vi "Private Global.vi"() -> ()   [LabVIEW 2016, in "Constants.lvlib"]
uses:
  Constants.lvlib
  Typedef/Constants.ctl
  <vilib>/Rock Robotics/SystemInterfaces/DIO/FPGA_DIOPWMChannel.ctl
  <vilib>/Rock Robotics/WPI/Joystick/WPI_JoystickDeviceEnum.ctl
  <vilib>/Rock Robotics/SystemInterfaces/DIO/FPGA_DIOChannel.ctl
  <vilib>/Rock Robotics/SystemInterfaces/spilib/spi_bus.ctl
  <vilib>/Rock Robotics/SystemInterfaces/AI/FPGA_AIChannel.ctl
  <vilib>/Rock Robotics/WPI/Solenoid/WPI_SolenoidChannel.ctl
panel:
  in  "Constants":T1={"Port Layout"={"RightMotorInverted"=FALSE, "LeftMotorInverted"=TRUE, "Left Motors"=enum."PWM 1", "Right Motors"=enum."PWM 0", "Auton List"=["None", "Score Gear Boiler Side", "Score Gear Boiler Side and Shoot", "Score Gear Hopper Side", "Score Gear Center"], "XBOX Port"=enum."USB 0", "Encoder L A"=enum."DIO 0", "Encoder L B"=enum."DIO 1", "Encoder R A"=enum."DIO 2", "Encoder R B"=enum."DIO 3", "L Encoder Inverse"=FALSE, "R Encoder Inverse"=TRUE, "Drive Distance per Count"=0.0490874, "Gyro Bus"=enum."SPI On-Board, CS0", "Fuel Roller 1"=enum."PWM 4", "Front Roller"=enum."PWM 3", "Gear Flipper"=enum."PWM 2", "Climber 1"=enum."PWM 7", "Fuel Roller Invert"=FALSE, "Front Roller Invert"=TRUE, "Gear Flipper Invert"=TRUE, "Climber Invert"=FALSE, "PCM"=1, "Fuel Roller 2"=enum."PWM 5", "Gear Sensor"=enum."AI 0", "Gear Release Fwd"=enum."Solenoid 3", "Gear Release Rvrs"=enum."Solenoid 2", "Fuel Arm Fwd"=enum."Solenoid 4", "Fuel Arm Rvrs"=enum."Solenoid 5", "Shifter Fwrd"=enum."Solenoid 0", "Shifter Rvrs"=enum."Solenoid 1", "Climber 2"=enum."PWM 6", "PDP"=60, "Shooter Front Channel"=3, "Shooter Rear Channel"=4, "Shooter Feed Channel"=5, "Camera Servo"=enum."PWM 8", "Gear Servo"=enum."PWM 9", "Gear Puncher Fwrd"=enum."Solenoid 6", "Gear Puncher Rvrs"=enum."Solenoid 7", "Shooter Inverse"=FALSE, "Ring Light Switch"=enum."DIO 4"}, "Drive Constants"={"Wheelbase In."=28.0, "Max Velocity (In/sec)"=50.0, "Max Accel (In/sec^2)"=50.0, "Max Jerk (In/sec^3)"=500.0, "Path dt"=0.005, "Path Sample Count"=10000, "Deadband"=0.2}, "Arm System"={"Front Roller Gear Speed"=-1.0, "Front Roller Fuel Speed"=1.0, "Gear Flipper Speed"=1.0, "Fuel Roller Speed"=1.0, "Gear Release Wait (ms)"=400, "Gear Sensor Threshold"=0.7, "Flappy Open Angle"=0, "Flappy Close Angle"=230, "Ramp Rate (EGU/min)"=150.0}, "Shooter"={"Shooter Wheels"={"P"=0.16, "I"=0.0015, "D"=10.0, "F"=0.065, "IZone"=2000.0}, "Feeder"={"P"=0.0, "I"=0.0, "D"=0.0, "F"=0.0, "IZone"=0.0}, "Front Shooter RPM"=5000.0, "Rear Shooter RPM"=4000.0, "Agitator Speed"=0.0, "Feeder Speed"=0.8, "Shooter CPR"=1024, "Feeder CPR"=0}, "Vision"={"High Goal Height (in.)"=78.0, "Low Goal Height (in.)"=13.5, "Camera Height High (in.)"=22.25, "Camera Height Low (in.)"=20.5, "Servo Pitch Gear (deg)"=-29.0, "Camera Yaw (deg)"=0.0, "Servo Gear"=0, "Servo Boiler"=205, "Servo Pitch Boiler (deg)"=0.0}}
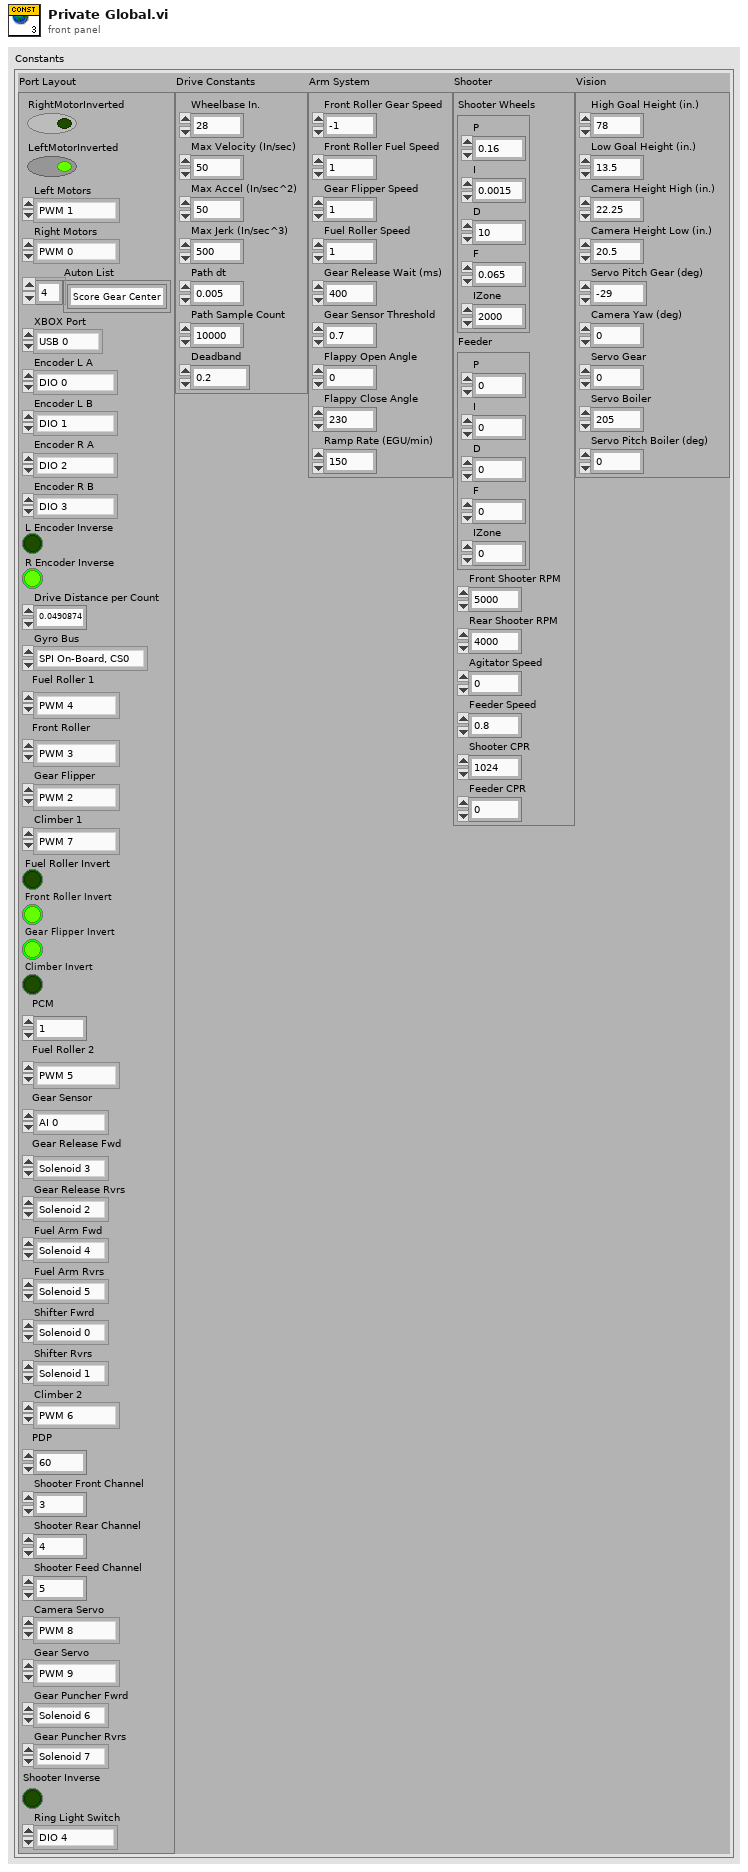
[diagram p1: front panel]
types:
  T1 = typedef "Constants.lvlib/Constants.ctl" = cluster{"Port Layout":cluster{"RightMotorInverted":bool, "LeftMotorInverted":bool, "Left Motors":T2, "Right Motors":T2, "Auton List":string[], "XBOX Port":T3, "Encoder L A":T4, "Encoder L B":T4, "Encoder R A":T4, "Encoder R B":T4, "L Encoder Inverse":bool, "R Encoder Inverse":bool, "Drive Distance per Count":dbl, "Gyro Bus":T5, "Fuel Roller 1":T2, "Front Roller":T2, "Gear Flipper":T2, "Climber 1":T2, "Fuel Roller Invert":bool, "Front Roller Invert":bool, "Gear Flipper Invert":bool, "Climber Invert":bool, "PCM":u8, "Fuel Roller 2":T2, "Gear Sensor":T6, "Gear Release Fwd":T7, "Gear Release Rvrs":T7, "Fuel Arm Fwd":T7, "Fuel Arm Rvrs":T7, "Shifter Fwrd":T7, "Shifter Rvrs":T7, "Climber 2":T2, "PDP":u8, "Shooter Front Channel":u8, "Shooter Rear Channel":u8, "Shooter Feed Channel":u8, "Camera Servo":T2, "Gear Servo":T2, "Gear Puncher Fwrd":T7, "Gear Puncher Rvrs":T7, "Shooter Inverse":bool, "Ring Light Switch":T4}, "Drive Constants":cluster{"Wheelbase In.":dbl, "Max Velocity (In/sec)":dbl, "Max Accel (In/sec^2)":dbl, "Max Jerk (In/sec^3)":dbl, "Path dt":dbl, "Path Sample Count":i32, "Deadband":dbl}, "Arm System":cluster{"Front Roller Gear Speed":dbl, "Front Roller Fuel Speed":dbl, "Gear Flipper Speed":dbl, "Fuel Roller Speed":dbl, "Gear Release Wait (ms)":i32, "Gear Sensor Threshold":dbl, "Flappy Open Angle":i32, "Flappy Close Angle":i32, "Ramp Rate (EGU/min)":dbl}, "Shooter":cluster{"Shooter Wheels":cluster{"P":dbl, "I":dbl, "D":dbl, "F":dbl, "IZone":dbl}, "Feeder":cluster{"P":dbl, "I":dbl, "D":dbl, "F":dbl, "IZone":dbl}, "Front Shooter RPM":dbl, "Rear Shooter RPM":dbl, "Agitator Speed":dbl, "Feeder Speed":dbl, "Shooter CPR":u32, "Feeder CPR":u32}, "Vision":cluster{"High Goal Height (in.)":dbl, "Low Goal Height (in.)":dbl, "Camera Height High (in.)":dbl, "Camera Height Low (in.)":dbl, "Servo Pitch Gear (deg)":dbl, "Camera Yaw (deg)":dbl, "Servo Gear":i32, "Servo Boiler":i32, "Servo Pitch Boiler (deg)":dbl}}
  T2 = typedef "FPGA_DIOPWMChannel.ctl" = enum8{"PWM 0", "PWM 1", "PWM 2", "PWM 3", "PWM 4", "PWM 5", "PWM 6", "PWM 7", "PWM 8", "PWM 9", "PWM MXP 0", "PWM MXP 1", "PWM MXP 2", "PWM MXP 3", "PWM MXP 4", "PWM MXP 5", "PWM MXP 6", "PWM MXP 7", "PWM MXP 8", "PWM MXP 9", "Invalid"}
  T3 = typedef "WPI_JoystickDeviceEnum.ctl" = enum16{"USB 0", "USB 1", "USB 2", "USB 3", "USB 4", "USB 5"}
  T4 = typedef "FPGA_DIOChannel.ctl" = enum8{"DIO 0", "DIO 1", "DIO 2", "DIO 3", "DIO 4", "DIO 5", "DIO 6", "DIO 7", "DIO 8", "DIO 9", "DIO MXP 0", "DIO MXP 1", "DIO MXP 2", "DIO MXP 3", "DIO MXP 4", "DIO MXP 5", "DIO MXP 6", "DIO MXP 7", "DIO MXP 8", "DIO MXP 9", "DIO MXP 10", "DIO MXP 11", "DIO MXP 12", "DIO MXP 13", "DIO MXP 14", "DIO MXP 15", "SPI Port CS1", "SPI Port CS2", "SPI Port CS3", "SPI Port MISO", "SPI Port MOSI", "Invalid"}
  T5 = typedef "spi_bus.ctl" = enum16{"SPI On-Board, CS0", "SPI On-Board, CS1", "SPI On-Board, CS2", "SPI On-Board, CS3", "SPI MXP", "Invalid"}
  T6 = typedef "FPGA_AIChannel.ctl" = enum8{"AI 0", "AI 1", "AI 2", "AI 3", "AI MXP 0", "AI MXP 1", "AI MXP 2", "AI MXP 3", "Invalid"}
  T7 = typedef "WPI_SolenoidChannel.ctl" = enum8{"Solenoid 0", "Solenoid 1", "Solenoid 2", "Solenoid 3", "Solenoid 4", "Solenoid 5", "Solenoid 6", "Solenoid 7", "Invalid"}
diagram:
